vi "LEP_RV_BuildSpec_DebugOptionsDlg.vi"(8 "error in (no error)":errorcluster, 10 "page sync rendezvous":T2, 11 "Close Event":refnum<user-event>) -> ()   [LabVIEW 2011]
doc: "Specifies advanced code generation options."
uses:
  resource/dialog/PreferencesDialog/optionsFrame_EventData1.ctl
  resource/dialog/PreferencesDialog/optionsFrame_PageInitData.ctl
panel:
  out "Build settings conflicts":i32(listbox)=1
  in  "Debugging mode":enum32{"Serial port", "TCP port", "USB JTAG"}(radio)
  in  "Enable profile information":bool
  in  "Page VI Init Data":T1
  in  "error msg format string":string="There was a problem applying the options from the %s category. The error message is \"%s.\""
  # "Build options"
  # "Debug options"
  # "Memory options"
  # "Debugging Mode"
  # "Good performance, additional code overhead;\nRequires serial cable connection between target and PC"
  # "Better performance, additional code overhead;\nRequires ethernet connection between target and PC"
  # "Best performance, no code overhead;\nNo additional cable needed"
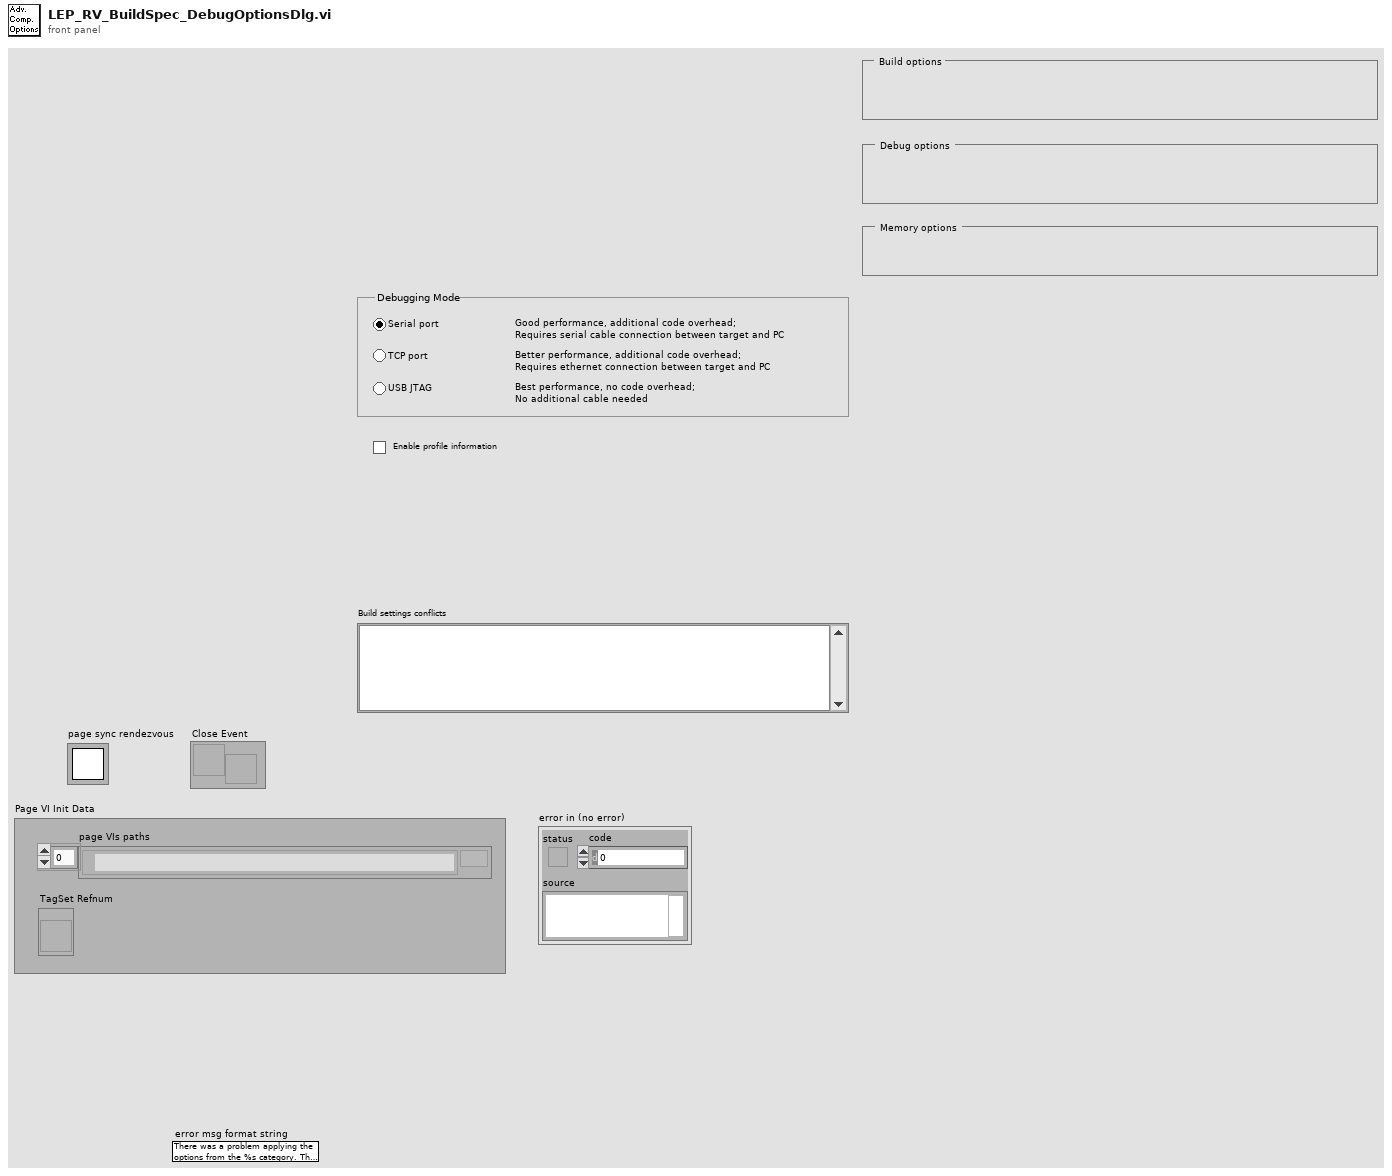
[diagram p1: front panel]
types:
  T1 = typedef "optionsFrame_PageInitData.ctl" = cluster{"page VIs paths":path[], "TagSet Refnum":refnum<vi>}
  T2 = typedef "Rendezvous RefNum" = refnum<k1>
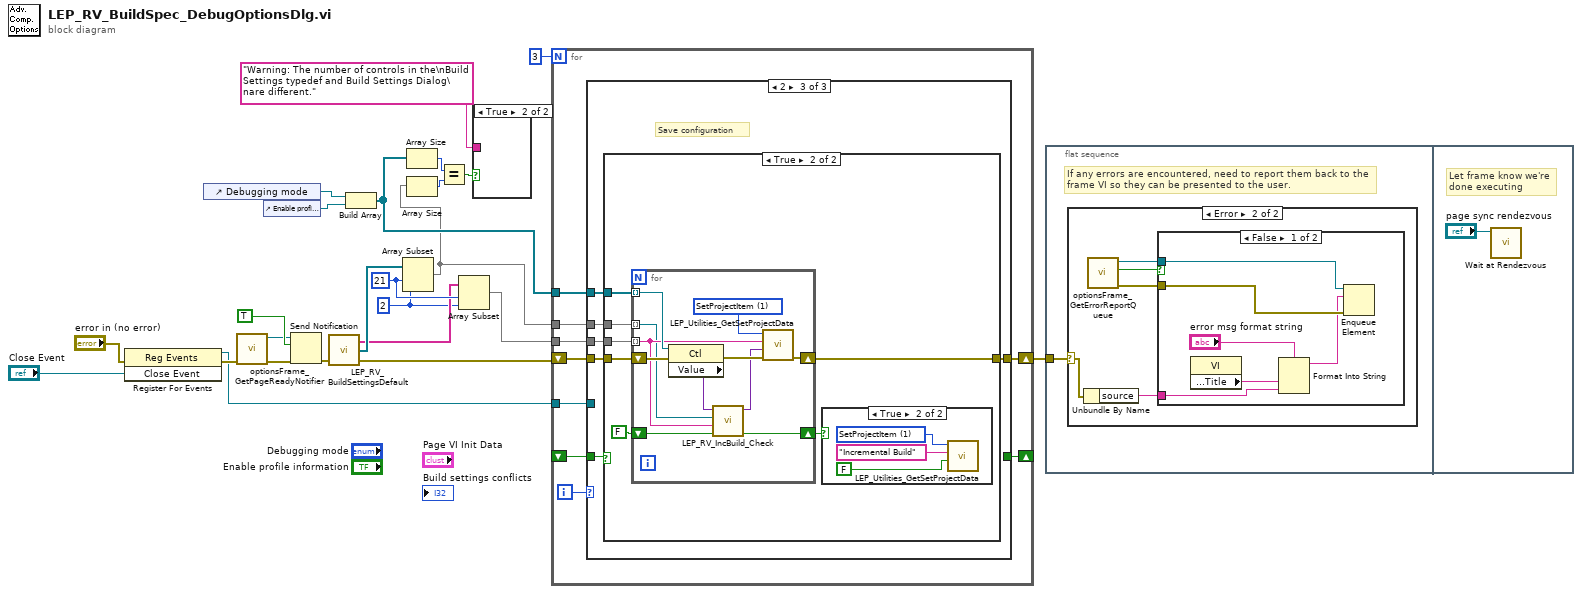
[diagram p0: block diagram]
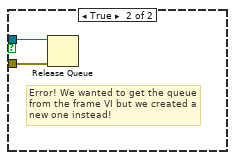
[diagram p3: hidden frame]
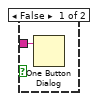
[diagram p4: hidden frame]
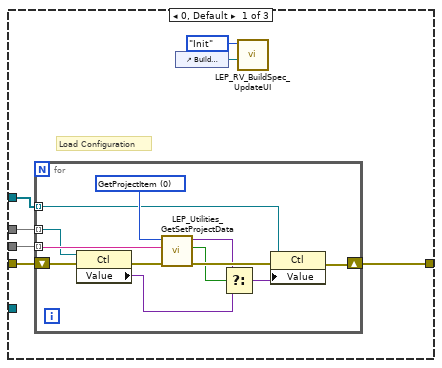
[diagram p5: hidden frame]
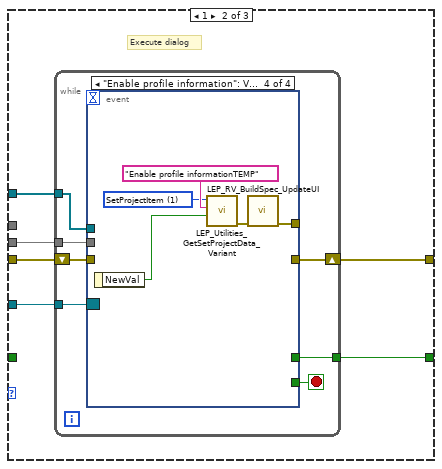
[diagram p6: hidden frame]
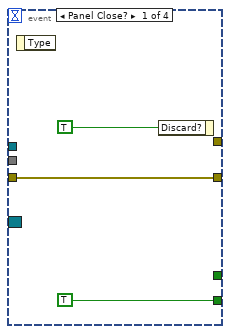
[diagram p7: hidden frame]
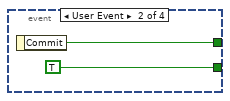
[diagram p8: hidden frame]
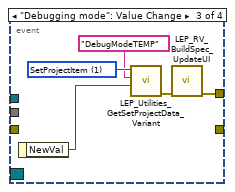
[diagram p9: hidden frame]
diagram:
  w4 = 2 ("length")
  w7 = 21 ("index")
  n1 = register-events(error in="error in (no error)", "Close Event") -> (reference out=w10:refnum<event-registration>, error out=w13:errorcluster)  [unwired: 1 in]
  n2 = control-ref of="Debugging mode"() -> (w3:refnum<vi>)
  n3 = call "optionsFrame_GetPageReadyNotifier.vi"("error in (no error)"=w13) -> ("error out"=w12:errorcluster, "notifier out"=w14:refnum<notifier>)  [unwired: 9 out]
  n4 = control-ref of="Enable profile information"() -> (w9:refnum<vi>)
  n5 = Send Notification(notification=TRUE, notifier=w14, error in (no error)=w12) -> (error out=w11:errorcluster)  [unwired: 1 out]
  n6 = call "LEP_RV_BuildSettingsDefault.vi"("error in (no error)"=w11) -> ("error out"=w23:errorcluster, "Default Values"=w8:refnum<vi>[], "Attribute Name"=w6:string[])  [unwired: 2 out]
  n7 = Build Array(w3, w9) -> (w19:refnum<vi>[])
  n8 = Array Subset(array=w8, index=w7, length=w4) -> (w2:refnum<vi>[])
  n9 = Array Size(array=w19) -> (size(s)=w21:i32)
  n10 = Array Size(array=w2) -> (size(s)=w22:i32)
  n11 = Equal?(x=w21, y=w22) -> (x = y?=w20:bool)
  n12 = Array Subset(array=w6, index=w7, length=w4) -> (w5:string[])
  n13 = case shown="True" w20 {
    tunnel: "Warning: The number of controls in the\nBuild Settings typedef and Build Settings Dialog\nare different." -> [w25 _]
    frame False {
      n14 = One Button Dialog(message=w25) -> ()  [unwired: 2 out]
    }
    frame True {
    }
  }
  n15 = for {
    N: 3 -> [_]
    shift-right: [w32] -> w1
    shift-left: w23 -> [w33]
    shift-right: [w31] -> _
    shift-left: _ -> [w30]
    tunnel: w19 -> [w29]
    tunnel: w5 -> [w28]
    tunnel: w2 -> [w27]
    tunnel: w10 -> [w26]
    i -> [w34]
    n16 = case shown="2" w34 {
      tunnel: w33 -> [w40 w59 w86]
      tunnel: [w37 w58 w85] -> w32
      tunnel: [_ w57 _] -> w31
      tunnel: w30 -> [_ _ w87]
      tunnel: w29 -> [w41 w55 w83]
      tunnel: w28 -> [w39 w56 w84]
      tunnel: w27 -> [w38 _ w82]
      tunnel: w26 -> [_ w54 _]
      frame 0, Default {
        # "Load Configuration"
        n17 = for {
          tunnel: w41 -> [w42] mode=indexing
          shift-right: [w51] -> w37
          shift-left: w40 -> [w49]
          tunnel: w39 -> [w50] mode=indexing
          tunnel: w38 -> [w47] mode=indexing
          w53 = u16 0 items=["GetProjectItem", "SetProjectItem"] ("Command")
          n18 = property class="Ctl"(reference=w47, error in=w49) -> (error out=w48:errorcluster, "Value"=w43:variant)  [unwired: 1 out]
          n19 = call-poly <vilib>:"LEP_Utilities_GetSetProjectData.vi"("error in"=w48, "ItemName"=w50, "Command"=w53) -> ("error out"=w52:errorcluster, "Found/Replaced?"=w44:bool, "Variant Out"=w45:variant)  [unwired: 2 in, 4 out]
          n20 = Select(t=w45, s=w44, f=w43) -> (s? t:f=w46:variant)
          n21 = property class="Ctl"(reference=w42, error in=w52, "Value"=w46) -> (error out=w51:errorcluster)  [unwired: 1 out]
        }
        n22 = control-ref of="Build settings conflicts"() -> (w35:refnum<vi>)
        n23 = call "LEP_RV_BuildSpec_UpdateUI.vi"("Build conflicts ref"=w35, "Action"=enum16{"Init", "UpdateUI"}."Init") -> ()  [unwired: 2 in, 8 out]
      }
      frame 1 {
        # "Execute dialog"
        n24 = while {
          shift-right: [w65] -> w58
          shift-left: w59 -> [w66]
          tunnel: [w64] -> w57
          tunnel: w56 -> [w62]
          tunnel: w55 -> [w61]
          tunnel: w54 -> [w60]
          stop <- w63 stop-if-true
          n25 = event shown="[3] \"Enable profile information\": Value Change" {
            selector: w60 -> [_ _ _ _]
            dyn-events: _ -> [_ _ _ _]
            timeout: _ -> [_ _ _ _]
            tunnel: w66 -> [w68 _ _ _]
            tunnel: [w68 _ _ _] -> w65
            tunnel: [_ w70 _ _] -> w64
            tunnel: [TRUE TRUE ("Cancel") _ _] -> w63
            tunnel: w62 -> [_ _ _ _]
            tunnel: w61 -> [_ _ _ _]
            tunnel: [_ _ w74 w78] -> _
            event Panel Close? {
              n26 = event-data() -> ()  [unwired: 2 out]
              n27 = event-data("Discard?"=TRUE) -> ()  [unwired: 1 in, 1 out]
            }
            event User Event {
              n28 = event-data() -> ("Commit"=w70:bool)  [unwired: 1 out]
            }
            event "Debugging mode": Value Change {
              w75 = u16 1 items=["GetProjectItem", "SetProjectItem"] ("Command")
              n29 = event-data() -> ("NewVal"=w76:enum32{"Serial port", "TCP port", "USB JTAG"})  [unwired: 1 out]
              n30 = call <vilib>:"LEP_Utilities_GetSetProjectData_Variant.vi"("Variant In"=w76, "ItemName"="DebugModeTEMP", "Command"=w75) -> ("error out"=w73:errorcluster)  [unwired: 2 in, 6 out]
              n31 = call "LEP_RV_BuildSpec_UpdateUI.vi"("error in (no error)"=w73) -> ("error out"=w74:errorcluster)  [unwired: 3 in, 7 out]
            }
            event "Enable profile information": Value Change {
              w80 = u16 1 items=["GetProjectItem", "SetProjectItem"] ("Command")
              n32 = event-data() -> ("NewVal"=w77:bool)  [unwired: 1 out]
              n33 = call <vilib>:"LEP_Utilities_GetSetProjectData_Variant.vi"("Variant In"=w77, "ItemName"="Enable profile informationTEMP", "Command"=w80) -> ("error out"=w79:errorcluster)  [unwired: 2 in, 6 out]
              n34 = call "LEP_RV_BuildSpec_UpdateUI.vi"("error in (no error)"=w79) -> ("error out"=w78:errorcluster)  [unwired: 3 in, 7 out]
            }
          }
        }
      }
      frame 2 {
        # "Save configuration"
        n35 = case shown="True" w87 {
          tunnel: w86 -> [w88 w95]
          tunnel: [w88 w92] -> w85
          tunnel: w84 -> [_ w94]
          tunnel: w83 -> [_ w93]
          tunnel: w82 -> [_ w91]
          frame False {
          }
          frame True {
            n36 = for {
              shift-right: [w106] -> w92
              shift-left: w95 -> [w108]
              tunnel: w94 -> [w102] mode=indexing
              tunnel: w93 -> [w105] mode=indexing
              tunnel: w91 -> [w101] mode=indexing
              shift-right: [w99] -> w89
              shift-left: FALSE -> [w100]
              w109 = u16 1 items=["GetProjectItem", "SetProjectItem"] ("Command")
              n37 = property class="Ctl"(reference=w105, error in=w108) -> (error out=w107:errorcluster, "Value"=w104:variant)  [unwired: 1 out]
              n38 = call "LEP_RV_IncBuild_Check.vi"("changed?"=w100, "attribute name"=w102, "default value"=w101, "control value"=w104) -> ("changed?"=w99:bool, "control value out"=w103:variant)  [unwired: 6 out]
              n39 = call-poly <vilib>:"LEP_Utilities_GetSetProjectData.vi"("error in"=w107, "Variant In"=w103, "ItemName"=w102, "Command"=w109) -> ("error out"=w106:errorcluster)  [unwired: 1 in, 6 out]
            }
            n40 = case shown="True" w89 {
              frame False {
              }
              frame True {
                w98 = u16 1 items=["GetProjectItem", "SetProjectItem"] ("Command")
                n41 = call-poly <vilib>:"LEP_Utilities_GetSetProjectData.vi"("Variant In"=FALSE, "ItemName"="Incremental Build", "Command"=w98) -> ()  [unwired: 2 in, 7 out]
              }
            }
          }
        }
      }
    }
  }
  n42 = flat-sequence {
    tunnel: w1 -> [w110]
    frame #0 {
      # "If any errors are encountered, need to report them back to the \nframe VI so they can be presented to the user."
      n43 = case shown="Error" w110 {
        selector: w110 -> [_ w112]
        frame No Error {
        }
        frame Error {
          n44 = Unbundle By Name(w112) -> ("source"=w111:string)
          n45 = call "optionsFrame_GetErrorReportQueue.vi"() -> ("error out"=w113:errorcluster, "created new?"=w115:bool, "queue out"=w114:refnum<queue>)  [unwired: 9 out]
          n46 = case shown="False" w115 {
            tunnel: w114 -> [w121 w123]
            tunnel: w113 -> [w120 w122]
            tunnel: w111 -> [w117 _]
            frame False {
              n47 = property class="VI"() -> ("Front Panel.Title"=w118:string)  [unwired: 2 in, 2 out]
              n48 = Format Into String(format string="error msg format string", w118, w117) -> (resulting string=w116:string)  [unwired: 2 in, 1 out]
              n49 = Enqueue Element(queue=w121, element=w116, error in (no error)=w120) -> ()  [unwired: 4 out]
            }
            frame True {
              # "Error! We wanted to get the queue\nfrom the frame VI but we created a\nnew one instead!"
              n50 = Release Queue(queue=w123, error in (no error)=w122) -> ()  [unwired: 4 out]
            }
          }
        }
      }
    }
    frame #1 {
      # "Let frame know we're \ndone executing"
      n51 = call <vilib>:"Wait at Rendezvous.vi"("rendezvous"="page sync rendezvous") -> ()  [unwired: 2 in, 5 out]
    }
  }
